vi "connect module disconnect.vi"() -> ()   [LabVIEW 2017]
uses:
  <instrlib>/Zurich Instruments LabOne/Public/ziTypeHandle.ctl
  <instrlib>/Zurich Instruments LabOne/Public/Modules/ziTypeModHandle.ctl
  <instrlib>/Zurich Instruments LabOne/Public/Modules/ziTypeModEnum.ctl
  <instrlib>/Zurich Instruments LabOne/Zurich Instruments LabOne.lvlib
panel:
  out "Handle Out":T1 {"Handle" format="0x%08x"; "Conn" format="0x%08x"}
  out "Finished?":bool
  out "Progress (unity)":dbl
  out "ModHandle":T2 {"ModHandle" format="0x%08x"; "Conn" format="0x%08x"}
  out "ModHandle Out":T2 {"ModHandle" format="0x%08x"; "Conn" format="0x%08x"}
  out "Handle":T1 {"Handle" format="0x%08x"; "Conn" format="0x%08x"}
  out "Selected Device":string
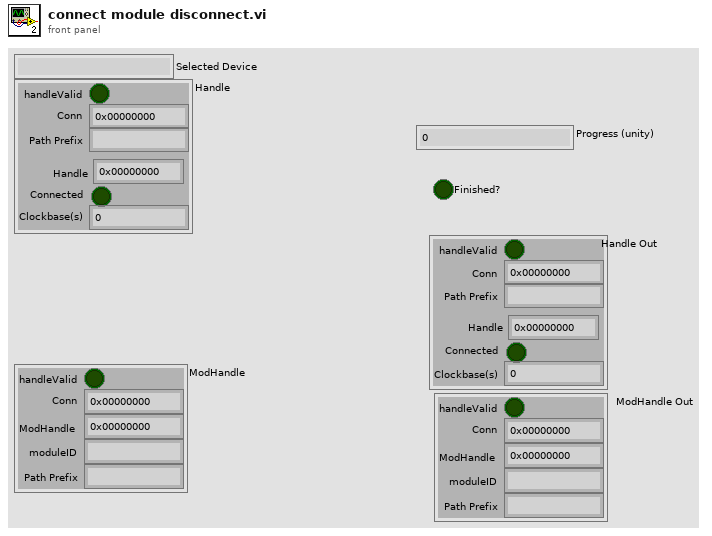
[diagram p1: front panel]
types:
  T1 = typedef "Zurich Instruments LabOne.lvlib/ziTypeHandle.ctl" = cluster{"handleValid":bool, "Conn":u64, "Path Prefix":string, "Handle":u64, "Connected":bool, "Clockbase(s)":dbl}
  T2 = typedef "Zurich Instruments LabOne.lvlib/ziTypeModHandle.ctl" = cluster{"handleValid":bool, "Conn":u64, "ModHandle":u64, "moduleID":string, "Path Prefix":string}
  T3 = typedef "Zurich Instruments LabOne.lvlib/ziTypeModEnum.ctl" = u16
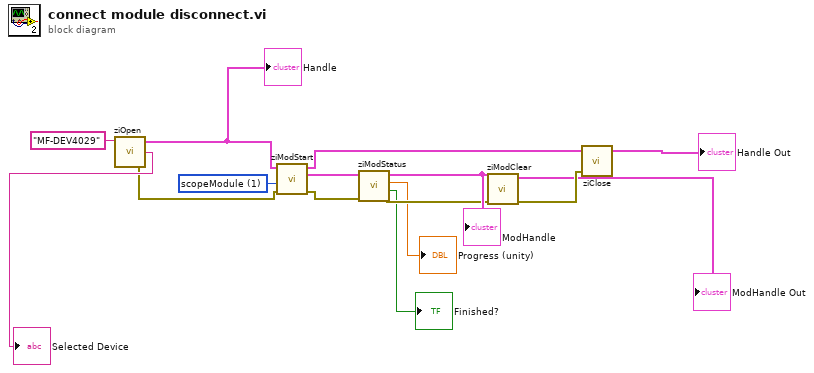
[diagram p0: block diagram]
diagram:
  w3 = T3 1 items=["sweep", "scopeModule", "dataAcquisitionModule", "pidAdvisor", "awgModule", "impedanceModule", "multiDeviceSyncModule", "zoomFFT", "trigger", "deviceSettings", "record", "precompensationAdvisor"] ("module Id")
  n1 = call <instrlib>:"ziOpen.vi"("Address"="MF-DEV4029") -> ("Error Out"=w2:errorcluster, "Selected Device"=→"Selected Device":string, "HandleOut"=w8:T1)  [unwired: 3 in]
  "Handle" <- w8
  n2 = call <instrlib>:"ziModStart.vi"("Error In"=w2, "module Id"=w3, "Handle In"=w8) -> ("Error Out"=w12:errorcluster, "ModHandle Out"=w13:T2, "Handle Out"=w1:T1)  [unwired: 6 in]
  n3 = call <instrlib>:"ziModStatus.vi"("Error In"=w12, "ModHandle IN"=w13) -> ("Error Out"=w10:errorcluster, "Finished?"=→"Finished?":bool, "Progress (unity)"=→"Progress (unity)":dbl, "ModHandle Out"=w11:T2)  [unwired: 5 in]
  "ModHandle" <- w11
  n4 = call <instrlib>:"ziModClear.vi"("Error In"=w10, "ziModHandle In"=w11) -> ("Error Out"=w9:errorcluster, "ModHandle Out"=→"ModHandle Out":T2)  [unwired: 7 in]
  n5 = call <instrlib>:"ziClose.vi"("Error In"=w9, "Handle In"=w1) -> ("Handle Out"=→"Handle Out":T1)  [unwired: 2 in, 1 out]
